vi "Find Visible.vi"(8 "Visible in":i16[][](array[numeric]), 11 "Height in":u8[][](array[numeric])) -> (0 "Visible in":i16[][](array[numeric]), 3 "Height out":u8[][](array[numeric]))   [LabVIEW 2021, in "d8.lvlib"]
uses:
  d8.lvlib
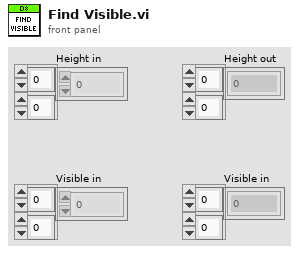
[diagram p1: front panel]
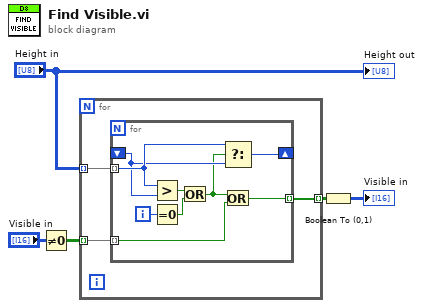
[diagram p0: block diagram]
diagram:
  n1 = Not Equal To 0?(x="Visible in") -> (x != 0?=w2:bool[][])
  n2 = for {
    tunnel: "Height in" -> [w8] mode=indexing
    tunnel: w2 -> [w7] mode=indexing
    tunnel: [w6] -> w4 mode=indexing
    n3 = for {
      tunnel: w8 -> [w13] mode=indexing
      shift-right: [w14] -> _
      shift-left: _ -> [w12]
      tunnel: [w10] -> w6 mode=indexing
      tunnel: w7 -> [w9] mode=indexing
      i -> [w16]
      n4 = Greater?(x=w13, y=w12) -> (0:w17:bool)
      n5 = Equal To 0?(x=w16) -> (x = 0?=w15:bool)
      n6 = Or(x=w17, y=w15) -> (x .or. y?=w11:bool)
      n7 = Select(t=w13, s=w11, f=w12) -> (s? t:f=w14:u8)
      n8 = Or(x=w11, y=w9) -> (x .or. y?=w10:bool)
    }
  }
  n9 = Boolean To (0,1)(Boolean=w4) -> (0, 1=→"Visible in":i16[][])
  "Height out" <- "Height in"
